vi "FPGACode_ReadWriteDigitalPorts.vi"(8 "EnableLoopBack":bool) -> (14 "Connector 0/DIOPORT2":u8, 15 "Connector 0/DIOPORT3":u8, 16 "Connector1/DIOPORT2":u8, 17 "Connector1/DIOPORT3":u8)   [LabVIEW 2023]
uses:
  <vilib>/rvi/Emulation/niFpgaGetClockAttributes.vi
  <vilib>/rvi/Emulation/niFpgaSctlEmulationGetInTimedLoop.vi
  <vilib>/rvi/Emulation/niFpgaEmulationReportErrorSimple.vi
  <vilib>/rvi/eio/common/nirviEmuTemplateMethod_errors.vi
  <vilib>/rvi/Emulation/niFpgaCriticalErrorInLSC.vi
  <vilib>/eio/EIONode/EIONode.xnode
panel:
  in  "Connector 0/DIOPORT0":u8
  in  "Connector1/DIOPORT1":u8
  in  "Connector1/DIOPORT0":u8
  in  "Connector 0/DIOPORT1":u8
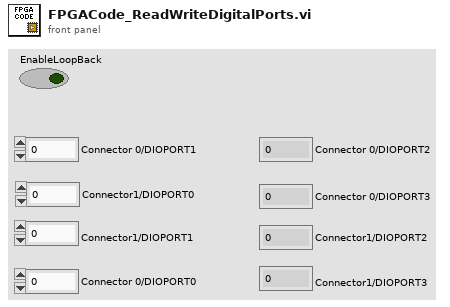
[diagram p1: front panel]
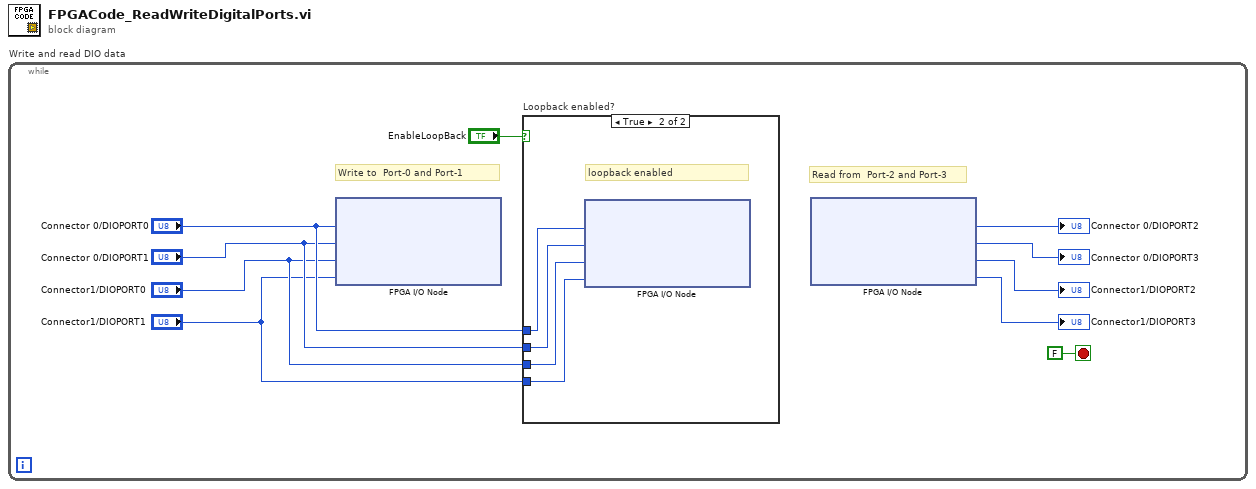
[diagram p0: block diagram]
diagram:
  n1 = while "Write and read DIO data" {
    stop <- FALSE stop-if-true
    # "Write to  Port-0 and Port-1"
    # "Read from  Port-2 and Port-3"
    n2 = xnode "FPGA I/O Node"("Connector0/DIOPORT0"="Connector 0/DIOPORT0", "Connector0/DIOPORT1"="Connector 0/DIOPORT1", "Connector1/DIOPORT0"="Connector1/DIOPORT0", "Connector1/DIOPORT1"="Connector1/DIOPORT1") -> ()  [unwired: 4 in, 4 out]
    n3 = case "Loopback enabled?" shown="True" "EnableLoopBack" {
      tunnel: "Connector 0/DIOPORT0" -> [_ w14]
      tunnel: "Connector 0/DIOPORT1" -> [_ w13]
      tunnel: "Connector1/DIOPORT0" -> [_ w12]
      tunnel: "Connector1/DIOPORT1" -> [_ w11]
      frame False {
      }
      frame True {
        # "loopback enabled"
        n4 = xnode "FPGA I/O Node"("Connector0/DIOPORT2"=w14, "Connector0/DIOPORT3"=w13, "Connector1/DIOPORT2"=w12, "Connector1/DIOPORT3"=w11) -> ()  [unwired: 4 in, 4 out]
      }
    }
    n5 = xnode "FPGA I/O Node"() -> ("Connector0/DIOPORT2"=→"Connector 0/DIOPORT2":u8, "Connector0/DIOPORT3"=→"Connector 0/DIOPORT3":u8, "Connector1/DIOPORT2"=→"Connector1/DIOPORT2":u8, "Connector1/DIOPORT3"=→"Connector1/DIOPORT3":u8)  [unwired: 4 in, 4 out]
  }
